vi "ArduinoLDCGUI.vi"() -> ()   [LabVIEW 2017]
doc: "Use this template to build a user interface event handler design pattern. Use this pattern for dialog boxes and other user interfaces. You also can create and execute user-defined events that the VI can handle the same way as user interface events."
uses:
  <vilib>/Utility/config.llb/Read Key (String).vi
  <vilib>/Utility/config.llb/Read Key (U32).vi
  <vilib>/Instr/_visa.llb/VISA Configure Serial Port (Instr).vi
  <vilib>/Utility/config.llb/Write Key (String).vi
  <vilib>/Utility/config.llb/Write Key (U32).vi
  <vilib>/Utility/config.llb/NI_LVConfig.lvlib
panel:
  in  "Log":bool
  out "time 2":string
  in  "Delay (s)":dbl=0.1 min=0.0 max=10.0 step=0.05
  in  "baud rate":u32(ring)=9600 items=["115200", "9600"]
  out "Version":string
  out "time":string
  out "450nm [mW]":dbl(slide) scale=0.1..100.0 scale format="%#1_1p"
  out "LaserOn":bool
  in  "DHT":bool
  out "Temp":string
  out "Humidity":string
  out "Serial":string
  in  "SetCurrent [mA]":i32(slide) min=0 max=120 step=2 scale=0.11..110.0
  out "405nm [mW]":dbl(slide) scale=0.1..100.0 scale format="%#1_1p"
  in  "ComPort":refnum<visa-resource-name>
  in  "Laser_On_Off":bool
  in  "stop":bool
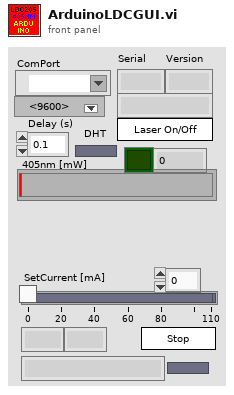
[diagram p1: front panel]
types:
  T1 = typedef "NI_LVConfig.lvlib/Config Data RefNum.ctl" = refnum<k1>
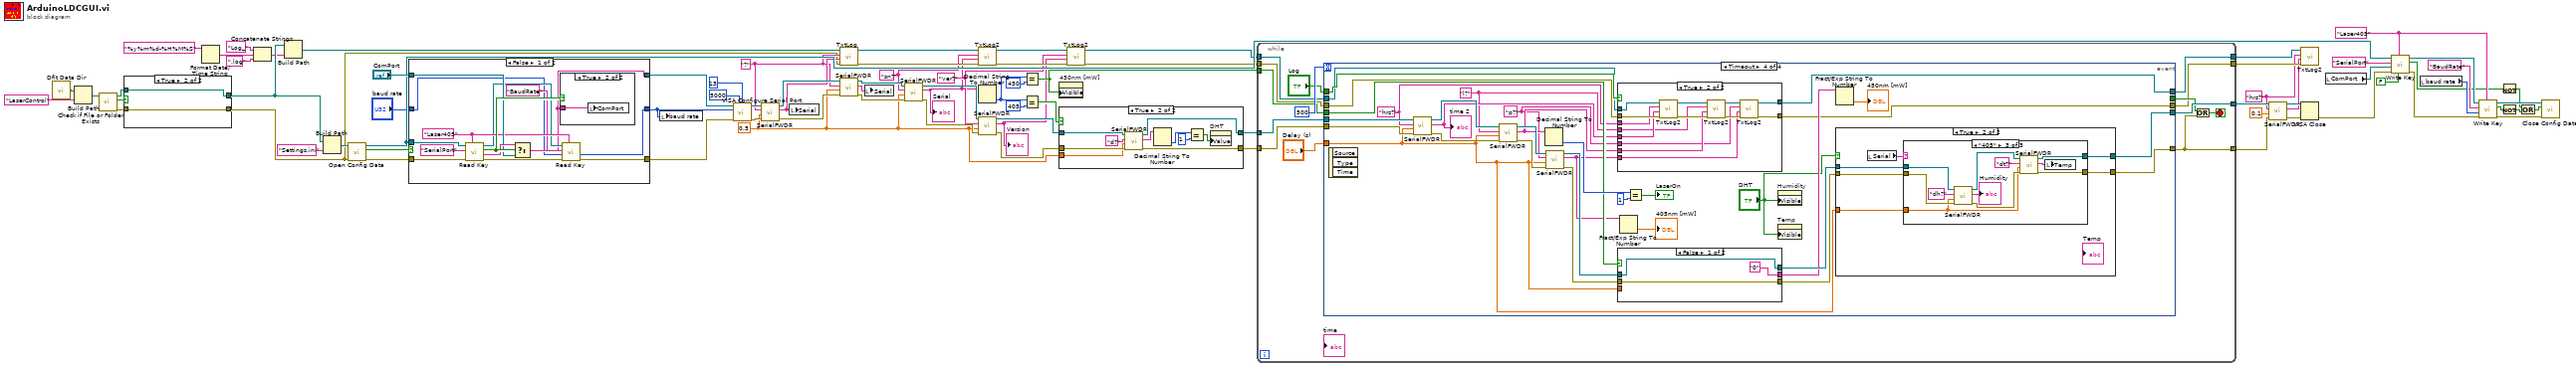
[diagram p0: block diagram]
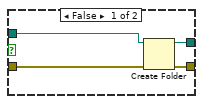
[diagram p4: hidden frame]
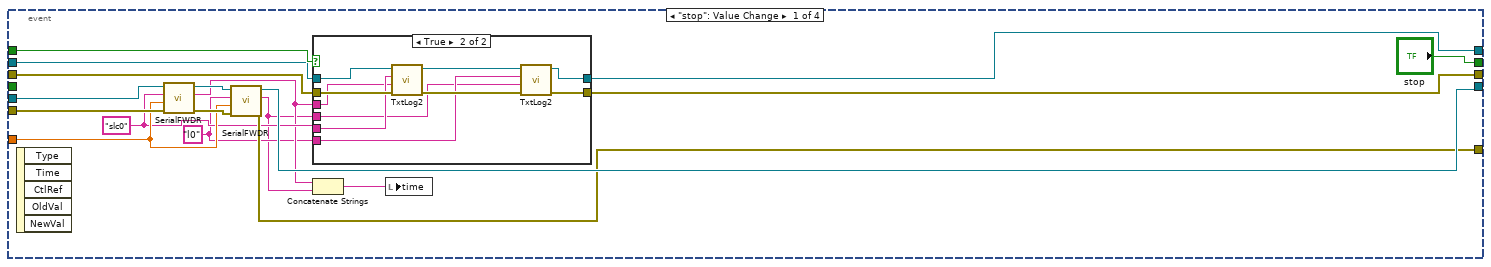
[diagram p6: hidden frame]
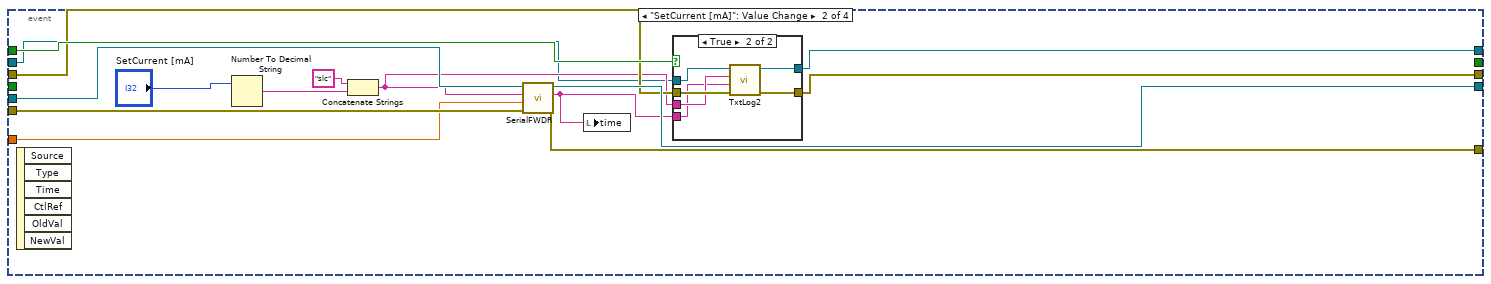
[diagram p8: hidden frame]
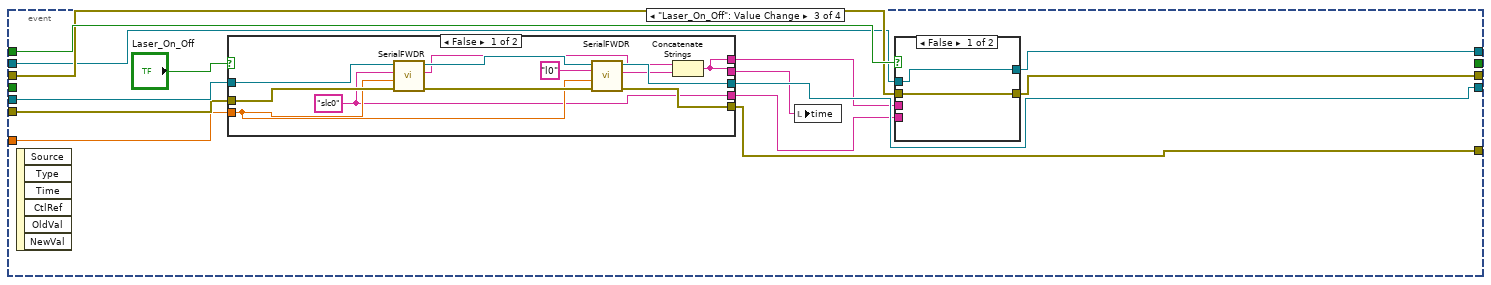
[diagram p10: hidden frame]
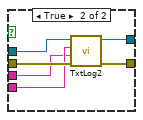
[diagram p11: hidden frame]
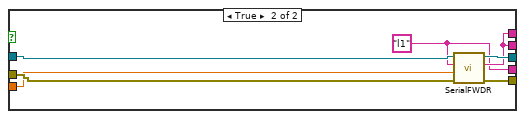
[diagram p12: hidden frame]
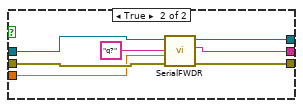
[diagram p14: hidden frame]
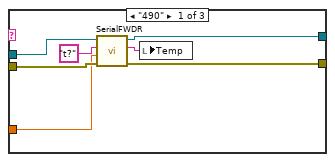
[diagram p16: hidden frame]
diagram:
  w2 = "hrs?" ("CommandString")
  w14 = "ver?" ("CommandString")
  w22 = "?" ("CommandString")
  w42 = 0.5 ("Delay Time (s)")
  w12 = "sn?" ("CommandString")
  w53 = "Laser405" ("section")
  n1 = call <vilib>:"Dflt Data Dir.vi"() -> ("App:Default Data Directory"=w78:path)
  n2 = Build Path(base path=w78, name or relative path="LaserControl") -> (appended path=w30:path)
  n3 = call <vilib>:"Check if File or Folder Exists.vi"("path"=w30) -> ("error out"=w73:errorcluster, "file or folder exists?"=w75:bool, "dup path"=w74:path)  [unwired: 8 in]
  n4 = case shown="True" w75 {
    tunnel: [w85 w88] -> w29
    tunnel: w74 -> [w86 w88]
    tunnel: w73 -> [w84 w87]
    tunnel: [w83 w87] -> w20
    frame False {
      n5 = Create Folder(path (use dialog)=w86, error in=w84) -> (created path=w85:path, error out=w83:errorcluster)  [unwired: 1 in, 1 out]
    }
    frame True {
    }
  }
  n6 = Format Date/Time String(time format string (%c)="%y%m%d-%H%M%S") -> (date/time string=w26:string)  [unwired: 2 in]
  n7 = Concatenate Strings("Log_" ("string"), w26, ".log" ("string")) -> (w24:string)
  n8 = Build Path(base path=w29, name or relative path=w24) -> (appended path=w21:path)
  n9 = Build Path(base path=w29, name or relative path="Settings.ini") -> (appended path=w76:path)
  n10 = call <vilib>:"Open Config Data.vi"("error in (no error)"=w20, "configuration file path"=w76) -> ("error out"=w71:errorcluster, "file created?"=w68:bool, "refnum"=w69:T1)  [unwired: 7 in]
  n11 = case shown="False" w68 {
    tunnel: "ComPort" -> [w98 w106]
    tunnel: w71 -> [w97 w105]
    tunnel: w69 -> [w99 _]
    tunnel: [w95 w105] -> w64
    tunnel: [w91 w106] -> w67
    tunnel: [w89 w104] -> w31
    tunnel: "baud rate" -> [w90 w104]
    frame False {
      w94 = "Laser405" ("section")
      n12 = call-poly <vilib>:"Read Key.vi"("section"=w94, "error in (no error)"=w97, "key"="SerialPort", "refnum"=w99) -> ("error out"=w96:errorcluster, "value"=w100:string, "found?"=w101:bool, "refnum out"=w92:T1)  [unwired: 4 in]
      n13 = Select(t=w100, s=w101, f=w98) -> (s? t:f=w91:string)
      n14 = case shown="True" w101 {
        tunnel: w91 -> [_ w103]
        frame False {
        }
        frame True {
          n15 = local write "ComPort"(w103) -> ()
        }
      }
      n16 = call-poly <vilib>:"Read Key.vi"("section"=w94, "error in (no error)"=w96, "default value"=w90, "key"="BaudRate", "refnum"=w92) -> ("error out"=w95:errorcluster, "value"=w89:u32)  [unwired: 3 in, 2 out]
    }
    frame True {
    }
  }
  n17 = local write "baud rate"(w31) -> ()
  n18 = call-poly "VISA Configure Serial Port"("VISA resource name"=w67, "timeout (10sec)"=u32 5000, "termination char\n(0xA = '\\n' = LF)"=u8 13 ("termination char\n(0xA = '\\n' = LF)"), "baud rate (9600)"=w31, "error in (no error)"=w64) -> ("VISA resource name out"=w62:refnum<visa-resource-name>, "error out"=w61:errorcluster)  [unwired: 9 in]
  n19 = call "SerialFWDR.vi"("error in (no error)"=w61, "Delay Time (s)"=w42, "CommandString"=w22, "VISA Refnum in"=w62) -> ("error out"=w57:errorcluster, "trimmed string"=w23:string, "VISA Refnum out"=w60:refnum<visa-resource-name>)  [unwired: 5 in]
  n20 = local write "Serial"(w23) -> ()
  n21 = call "TxtLog.vi"("error in (no error)"=w20, "trimmed string"=w23, "CommandString"=w22, "appended path"=w21) -> ("error out"=w19:errorcluster, "Byte Stream File out"=w18:refnum<file>)  [unwired: 6 in]
  n22 = call "SerialFWDR.vi"("error in (no error)"=w57, "Delay Time (s)"=w42, "CommandString"=w22, "VISA Refnum in"=w60) -> ("error out"=w56:errorcluster, "trimmed string"=w58:string, "VISA Refnum out"=w59:refnum<visa-resource-name>)  [unwired: 5 in]
  n23 = local write "Serial"(w58) -> ()
  n24 = call "SerialFWDR.vi"("error in (no error)"=w56, "Delay Time (s)"=w42, "CommandString"=w12, "VISA Refnum in"=w59) -> ("error out"=w46:errorcluster, "trimmed string"=w11:string, "VISA Refnum out"=w44:refnum<visa-resource-name>)  [unwired: 5 in]
  "Serial" <- w11
  n25 = call "TxtLog2.vi"("error in (no error)"=w19, "trimmed string"=w11, "CommandString"=w12, "Byte Stream File in"=w18) -> ("error out"=w16:errorcluster, "Byte Stream File out"=w17:refnum<file>)  [unwired: 6 in]
  n26 = Decimal String To Number(string=w11) -> (number=w40:i32)  [unwired: 2 in, 1 out]
  n27 = call "SerialFWDR.vi"("error in (no error)"=w46, "Delay Time (s)"=w42, "CommandString"=w14, "VISA Refnum in"=w44) -> ("error out"=w45:errorcluster, "trimmed string"=w13:string, "VISA Refnum out"=w43:refnum<visa-resource-name>)  [unwired: 5 in]
  "Version" <- w13
  n28 = Equal?(x=w40, y=450) -> (x = y?=w41:bool)
  n29 = Equal?(x=w40, y=405) -> (x = y?=w37:bool)
  n30 = property on="450nm [mW]" class="Slide (strict)"("Visible"=w41) -> ()  [unwired: 2 in, 2 out]
  n31 = case shown="True" w37 {
    tunnel: w45 -> [w107 w118]
    tunnel: [w107 w117] -> w82
    tunnel: w43 -> [w108 w115]
    tunnel: [w108 w116] -> w81
    tunnel: w42 -> [_ w113]
    frame False {
    }
    frame True {
      n32 = call "SerialFWDR.vi"("error in (no error)"=w118, "Delay Time (s)"=w113, "CommandString"="d?", "VISA Refnum in"=w115) -> ("error out"=w117:errorcluster, "trimmed string"=w110:string, "VISA Refnum out"=w116:refnum<visa-resource-name>)  [unwired: 5 in]
      n33 = Decimal String To Number(string=w110) -> (number=w111:i32)  [unwired: 2 in, 1 out]
      n34 = Equal?(x=w111, y=1) -> (x = y?=w109:bool)
      n35 = property on="DHT" class="Bool (strict)"("Value"=w109) -> ()  [unwired: 2 in, 2 out]
    }
  }
  n36 = call "TxtLog2.vi"("error in (no error)"=w16, "trimmed string"=w13, "CommandString"=w14, "Byte Stream File in"=w17) -> ("error out"=w15:errorcluster, "Byte Stream File out"=w10:refnum<file>)  [unwired: 6 in]
  n37 = while {
    tunnel: w81 -> [w131]
    tunnel: w82 -> [w130]
    tunnel: [w127] -> w7
    tunnel: [w132] -> w5
    tunnel: w41 -> [w125]
    tunnel: w15 -> [w122]
    tunnel: w10 -> [w121]
    tunnel: [w120] -> w9
    tunnel: [w119] -> w8
    stop <- w128 stop-if-true
    n38 = event shown="[3] Timeout" {
      selector: _ -> [_ _ _ _]
      dyn-events: _ -> [_ _ _ _]
      timeout: 500 -> [_ _ _ _]
      tunnel: ["stop" _ _ _] -> w126
      tunnel: [w148 w172 w196 w257] -> w127
      tunnel: w130 -> [w147 w173 w197 w255]
      tunnel: [w149 w174 w199 w258] -> w132
      tunnel: w131 -> [w145 w175 w198 w256]
      tunnel: w125 -> [_ _ _ w240]
      tunnel: "Delay (s)" -> [w142 w170 w193 w238]
      tunnel: "Log" -> [w136 w169 w192 w237]
      tunnel: w122 -> [w141 w168 w191 w236]
      tunnel: w121 -> [w135 w164 w187 w229]
      tunnel: [w133 w165 w188 w228] -> w120
      tunnel: [w134 w163 w186 w227] -> w119
      event "stop": Value Change {
        w140 = "slc0" ("CommandString")
        w138 = "l0" ("CommandString")
        n39 = event-data() -> ()  [unwired: 1 in, 5 out]
        n40 = call "SerialFWDR.vi"("error in (no error)"=w147, "Delay Time (s)"=w142, "CommandString"=w140, "VISA Refnum in"=w145) -> ("error out"=w146:errorcluster, "trimmed string"=w139:string, "VISA Refnum out"=w144:refnum<visa-resource-name>)  [unwired: 5 in]
        n41 = call "SerialFWDR.vi"("error in (no error)"=w146, "Delay Time (s)"=w142, "CommandString"=w138, "VISA Refnum in"=w144) -> ("error out"=w148:errorcluster, "trimmed string"=w137:string, "VISA Refnum out"=w149:refnum<visa-resource-name>)  [unwired: 5 in]
        n42 = case shown="True" w136 {
          tunnel: w141 -> [w152 w162]
          tunnel: w139 -> [_ w159]
          tunnel: w140 -> [_ w160]
          tunnel: w138 -> [_ w156]
          tunnel: w137 -> [_ w155]
          tunnel: w135 -> [w151 w161]
          tunnel: [w151 w154] -> w134
          tunnel: [w152 w153] -> w133
          frame False {
          }
          frame True {
            n43 = call "TxtLog2.vi"("error in (no error)"=w162, "trimmed string"=w159, "CommandString"=w160, "Byte Stream File in"=w161) -> ("error out"=w158:errorcluster, "Byte Stream File out"=w157:refnum<file>)  [unwired: 6 in]
            n44 = call "TxtLog2.vi"("error in (no error)"=w158, "trimmed string"=w155, "CommandString"=w156, "Byte Stream File in"=w157) -> ("error out"=w153:errorcluster, "Byte Stream File out"=w154:refnum<file>)  [unwired: 6 in]
          }
        }
        n45 = Concatenate Strings(w139, w137) -> (w143:string)
        n46 = local write "time"(w143) -> ()
      }
      event "SetCurrent [mA]": Value Change {
        n47 = event-data() -> ()  [unwired: 1 in, 6 out]
        n48 = Number To Decimal String(number="SetCurrent [mA]") -> (decimal integer string=w176:string)  [unwired: 1 in]
        n49 = Concatenate Strings("slc" ("string"), w176) -> (w167:string)
        n50 = call "SerialFWDR.vi"("error in (no error)"=w173, "Delay Time (s)"=w170, "CommandString"=w167, "VISA Refnum in"=w175) -> ("error out"=w172:errorcluster, "trimmed string"=w166:string, "VISA Refnum out"=w174:refnum<visa-resource-name>)  [unwired: 5 in]
        n51 = local write "time"(w166) -> ()
        n52 = case shown="True" w169 {
          tunnel: w168 -> [w178 w185]
          tunnel: w166 -> [_ w180]
          tunnel: w167 -> [_ w181]
          tunnel: [w178 w184] -> w165
          tunnel: w164 -> [w179 w183]
          tunnel: [w179 w182] -> w163
          frame False {
          }
          frame True {
            n53 = call "TxtLog2.vi"("error in (no error)"=w185, "trimmed string"=w180, "CommandString"=w181, "Byte Stream File in"=w183) -> ("error out"=w184:errorcluster, "Byte Stream File out"=w182:refnum<file>)  [unwired: 6 in]
          }
        }
      }
      event "Laser_On_Off": Value Change {
        n54 = event-data() -> ()  [unwired: 1 in, 6 out]
        n55 = case shown="False" "Laser_On_Off" {
          tunnel: [w219 w225] -> w199
          tunnel: w198 -> [w217 w226]
          tunnel: w197 -> [w215 w224]
          tunnel: [w218 w223] -> w196
          tunnel: [w208 w221] -> w194
          tunnel: w193 -> [w212 w222]
          tunnel: [w210 w220] -> w190
          tunnel: [w208 w221] -> w189
          frame False {
            w210 = "slc0" ("CommandString")
            n56 = call "SerialFWDR.vi"("error in (no error)"=w215, "Delay Time (s)"=w212, "CommandString"=w210, "VISA Refnum in"=w217) -> ("error out"=w214:errorcluster, "trimmed string"=w209:string, "VISA Refnum out"=w216:refnum<visa-resource-name>)  [unwired: 5 in]
            n57 = call "SerialFWDR.vi"("error in (no error)"=w214, "Delay Time (s)"=w212, "CommandString"="l0", "VISA Refnum in"=w216) -> ("error out"=w218:errorcluster, "trimmed string"=w213:string, "VISA Refnum out"=w219:refnum<visa-resource-name>)  [unwired: 5 in]
            n58 = Concatenate Strings(w209, w213) -> (w208:string)
          }
          frame True {
            w220 = "l1" ("CommandString")
            n59 = call "SerialFWDR.vi"("error in (no error)"=w224, "Delay Time (s)"=w222, "CommandString"=w220, "VISA Refnum in"=w226) -> ("error out"=w223:errorcluster, "trimmed string"=w221:string, "VISA Refnum out"=w225:refnum<visa-resource-name>)  [unwired: 5 in]
          }
        }
        n60 = local write "time"(w194) -> ()
        n61 = case shown="False" w192 {
          tunnel: w191 -> [w200 w207]
          tunnel: w190 -> [_ w203]
          tunnel: w189 -> [_ w202]
          tunnel: [w200 w206] -> w188
          tunnel: w187 -> [w201 w205]
          tunnel: [w201 w204] -> w186
          frame False {
          }
          frame True {
            n62 = call "TxtLog2.vi"("error in (no error)"=w207, "trimmed string"=w202, "CommandString"=w203, "Byte Stream File in"=w205) -> ("error out"=w206:errorcluster, "Byte Stream File out"=w204:refnum<file>)  [unwired: 6 in]
          }
        }
      }
      event Timeout {
        w231 = "p?" ("CommandString")
        w233 = "l?" ("CommandString")
        w235 = "hrs?" ("CommandString")
        n63 = event-data() -> ()  [unwired: 1 in, 3 out]
        n64 = call "SerialFWDR.vi"("error in (no error)"=w255, "Delay Time (s)"=w238, "CommandString"=w235, "VISA Refnum in"=w256) -> ("error out"=w253:errorcluster, "trimmed string"=w234:string, "VISA Refnum out"=w254:refnum<visa-resource-name>)  [unwired: 5 in]
        "time 2" <- w234
        n65 = call "SerialFWDR.vi"("error in (no error)"=w253, "Delay Time (s)"=w238, "CommandString"=w233, "VISA Refnum in"=w254) -> ("error out"=w248:errorcluster, "trimmed string"=w232:string, "VISA Refnum out"=w249:refnum<visa-resource-name>)  [unwired: 5 in]
        n66 = Decimal String To Number(string=w232) -> (number=w251:i32)  [unwired: 2 in, 1 out]
        n67 = call "SerialFWDR.vi"("error in (no error)"=w248, "Delay Time (s)"=w238, "CommandString"=w231, "VISA Refnum in"=w249) -> ("error out"=w247:errorcluster, "trimmed string"=w230:string, "VISA Refnum out"=w245:refnum<visa-resource-name>)  [unwired: 5 in]
        n68 = case shown="True" w237 {
          tunnel: w236 -> [w260 w274]
          tunnel: w235 -> [_ w272]
          tunnel: w234 -> [_ w273]
          tunnel: w233 -> [_ w264]
          tunnel: w232 -> [_ w263]
          tunnel: w231 -> [_ w261]
          tunnel: w230 -> [_ w262]
          tunnel: w229 -> [w259 w271]
          tunnel: [w260 w266] -> w228
          tunnel: [w259 w265] -> w227
          frame False {
          }
          frame True {
            n69 = call "TxtLog2.vi"("error in (no error)"=w274, "trimmed string"=w273, "CommandString"=w272, "Byte Stream File in"=w271) -> ("error out"=w268:errorcluster, "Byte Stream File out"=w270:refnum<file>)  [unwired: 6 in]
            n70 = call "TxtLog2.vi"("error in (no error)"=w268, "trimmed string"=w263, "CommandString"=w264, "Byte Stream File in"=w270) -> ("error out"=w267:errorcluster, "Byte Stream File out"=w269:refnum<file>)  [unwired: 6 in]
            n71 = call "TxtLog2.vi"("error in (no error)"=w267, "trimmed string"=w262, "CommandString"=w261, "Byte Stream File in"=w269) -> ("error out"=w266:errorcluster, "Byte Stream File out"=w265:refnum<file>)  [unwired: 6 in]
          }
        }
        n72 = case shown="False" w240 {
          tunnel: w247 -> [w277 w284]
          tunnel: [w277 w283] -> w246
          tunnel: w245 -> [w276 w282]
          tunnel: [w276 w281] -> w244
          tunnel: w238 -> [_ w280]
          tunnel: ["0" ("trimmed string") w278] -> w242
          frame False {
          }
          frame True {
            n73 = call "SerialFWDR.vi"("error in (no error)"=w284, "Delay Time (s)"=w280, "CommandString"="q?", "VISA Refnum in"=w282) -> ("error out"=w283:errorcluster, "trimmed string"=w278:string, "VISA Refnum out"=w281:refnum<visa-resource-name>)  [unwired: 5 in]
          }
        }
        n74 = Fract/Exp String To Number(string=w230) -> (number=→"405nm [mW]":dbl)  [unwired: 3 in, 1 out]
        n75 = Equal?(x=w251, y=1) -> (x = y?=→"LaserOn":bool)
        n76 = property on="Humidity" class="Str"("Visible"="DHT") -> ()  [unwired: 2 in, 2 out]
        n77 = property on="Temp" class="Str"("Visible"="DHT") -> ()  [unwired: 2 in, 2 out]
        n78 = Fract/Exp String To Number(string=w242) -> (number=→"450nm [mW]":dbl)  [unwired: 3 in, 1 out]
        n79 = case shown="True" "DHT" {
          tunnel: [w286 w289] -> w257
          tunnel: [w285 w291] -> w258
          tunnel: w244 -> [w285 w292]
          tunnel: w246 -> [w286 w290]
          tunnel: w238 -> [_ w287]
          frame False {
          }
          frame True {
            n80 = local read "Serial"() -> (w288:string)
            n81 = case shown="\"405\"" w288 {
              tunnel: w292 -> [w299 w301 w312]
              tunnel: [w298 w301 w310] -> w291
              tunnel: w290 -> [w297 w300 w309]
              tunnel: [w296 w300 w307] -> w289
              tunnel: w287 -> [w293 _ w302]
              frame "490" {
                n82 = call "SerialFWDR.vi"("error in (no error)"=w297, "Delay Time (s)"=w293, "CommandString"="t?", "VISA Refnum in"=w299) -> ("error out"=w296:errorcluster, "trimmed string"=w295:string, "VISA Refnum out"=w298:refnum<visa-resource-name>)  [unwired: 5 in]
                n83 = local write "Temp"(w295) -> ()
              }
              frame "False", Default {
              }
              frame "405" {
                n84 = call "SerialFWDR.vi"("error in (no error)"=w309, "Delay Time (s)"=w302, "CommandString"="dh?", "VISA Refnum in"=w312) -> ("error out"=w308:errorcluster, "trimmed string"=→"Humidity":string, "VISA Refnum out"=w311:refnum<visa-resource-name>)  [unwired: 5 in]
                n85 = call "SerialFWDR.vi"("error in (no error)"=w308, "Delay Time (s)"=w302, "CommandString"="dt?", "VISA Refnum in"=w311) -> ("error out"=w307:errorcluster, "trimmed string"=w303:string, "VISA Refnum out"=w310:refnum<visa-resource-name>)  [unwired: 5 in]
                n86 = local write "Temp"(w303) -> ()
              }
            }
          }
        }
      }
    }
    n87 = Or(x=w126, y=w127) -> (x .or. y?=w128:bool)
  }
  n88 = call "SerialFWDR.vi"("error in (no error)"=w7, "Delay Time (s)"=0.1, "CommandString"=w2, "VISA Refnum in"=w5) -> ("error out"=w6:errorcluster, "trimmed string"=w1:string, "VISA Refnum out"=w4:refnum<visa-resource-name>)  [unwired: 5 in]
  n89 = call "TxtLog2.vi"("error in (no error)"=w9, "trimmed string"=w1, "CommandString"=w2, "Byte Stream File in"=w8) -> ()  [unwired: 6 in, 2 out]
  n90 = VISA Close(VISA resource name=w4, error in (no error)=w6) -> (error out=w63:errorcluster)
  n91 = local read "ComPort"() -> (w79:refnum<visa-resource-name>)
  n92 = call-poly <vilib>:"Write Key.vi"("write raw string? (F)"=FALSE, "section"=w53, "error in (no error)"=w63, "value"=w79, "key"="SerialPort", "refnum"=w69) -> ("error out"=w55:errorcluster, "found?"=w36:bool, "refnum out"=w54:T1)  [unwired: 3 in]
  n93 = local read "baud rate"() -> (w47:u32)
  n94 = call-poly <vilib>:"Write Key.vi"("section"=w53, "error in (no error)"=w55, "value"=w47, "key"="BaudRate", "refnum"=w54) -> ("error out"=w49:errorcluster, "found?"=w35:bool, "refnum out"=w50:T1)  [unwired: 4 in]
  n95 = Not(x=w36) -> (.not. x?=w34:bool)
  n96 = Not(x=w35) -> (.not. x?=w33:bool)
  n97 = Or(x=w34, y=w33) -> (x .or. y?=w32:bool)
  n98 = call <vilib>:"Close Config Data.vi"("error in (no error)"=w49, "write file if changed (T)"=w32, "refnum"=w50) -> ()  [unwired: 7 in, 2 out]
